vi "test2-SyncMessageWithError.vi"(8 "error in (no error)":errorcluster, 11 "TestCase in":refnum<class "testcase-CSMMessage.lvclass">) -> (0 "error out":errorcluster, 3 "TestCase out":refnum<class "testcase-CSMMessage.lvclass">)   [LabVIEW 2017, in "testcase-CSMMessage.lvclass"]
uses:
  testcase-CSMMessage.lvclass
  1ed8f569-7b65-4950-a766-51d9a6509acb.vi
  src/user.lib/_NEVSTOP/Communicable State Machine(CSM)/AdvanceAPI/CSM - Make String Arguments Safe.vi
  src/user.lib/_NEVSTOP/Communicable State Machine(CSM)/AdvanceAPI/CSM - Keywords.vi
  <vilib>/addons/_JKI Toolkits/VI Tester/TestCase.llb/TestCase.lvclass
  src/user.lib/_NEVSTOP/Communicable State Machine(CSM)/Communicable State Machine.lvlib
  C:/Program Files (x86)/National Instruments/LabVIEW 2017/vi.lib/addons/_JKI Toolkits/VI Tester/TestCase.llb/TestCase.lvclass
panel:
  out "Loopcount":i32
  out "concatenated string":string
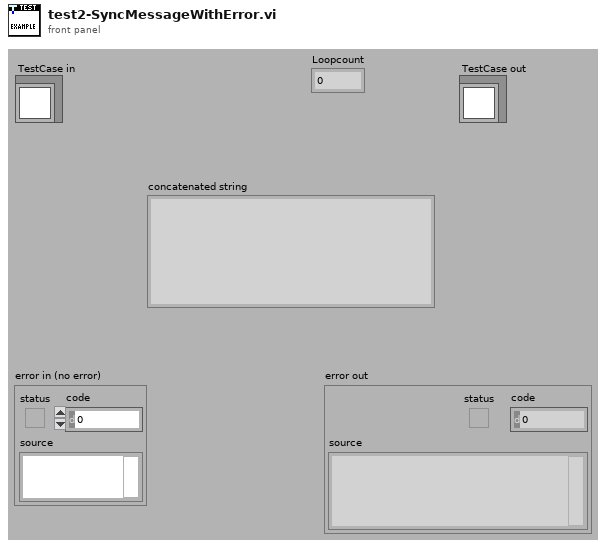
[diagram p1: front panel]
types:
  T1 = cluster{"Arguments":string, "Response":string, "error":errorcluster}
  T2 = cluster{"status":bool, "code":bool, "source":bool}
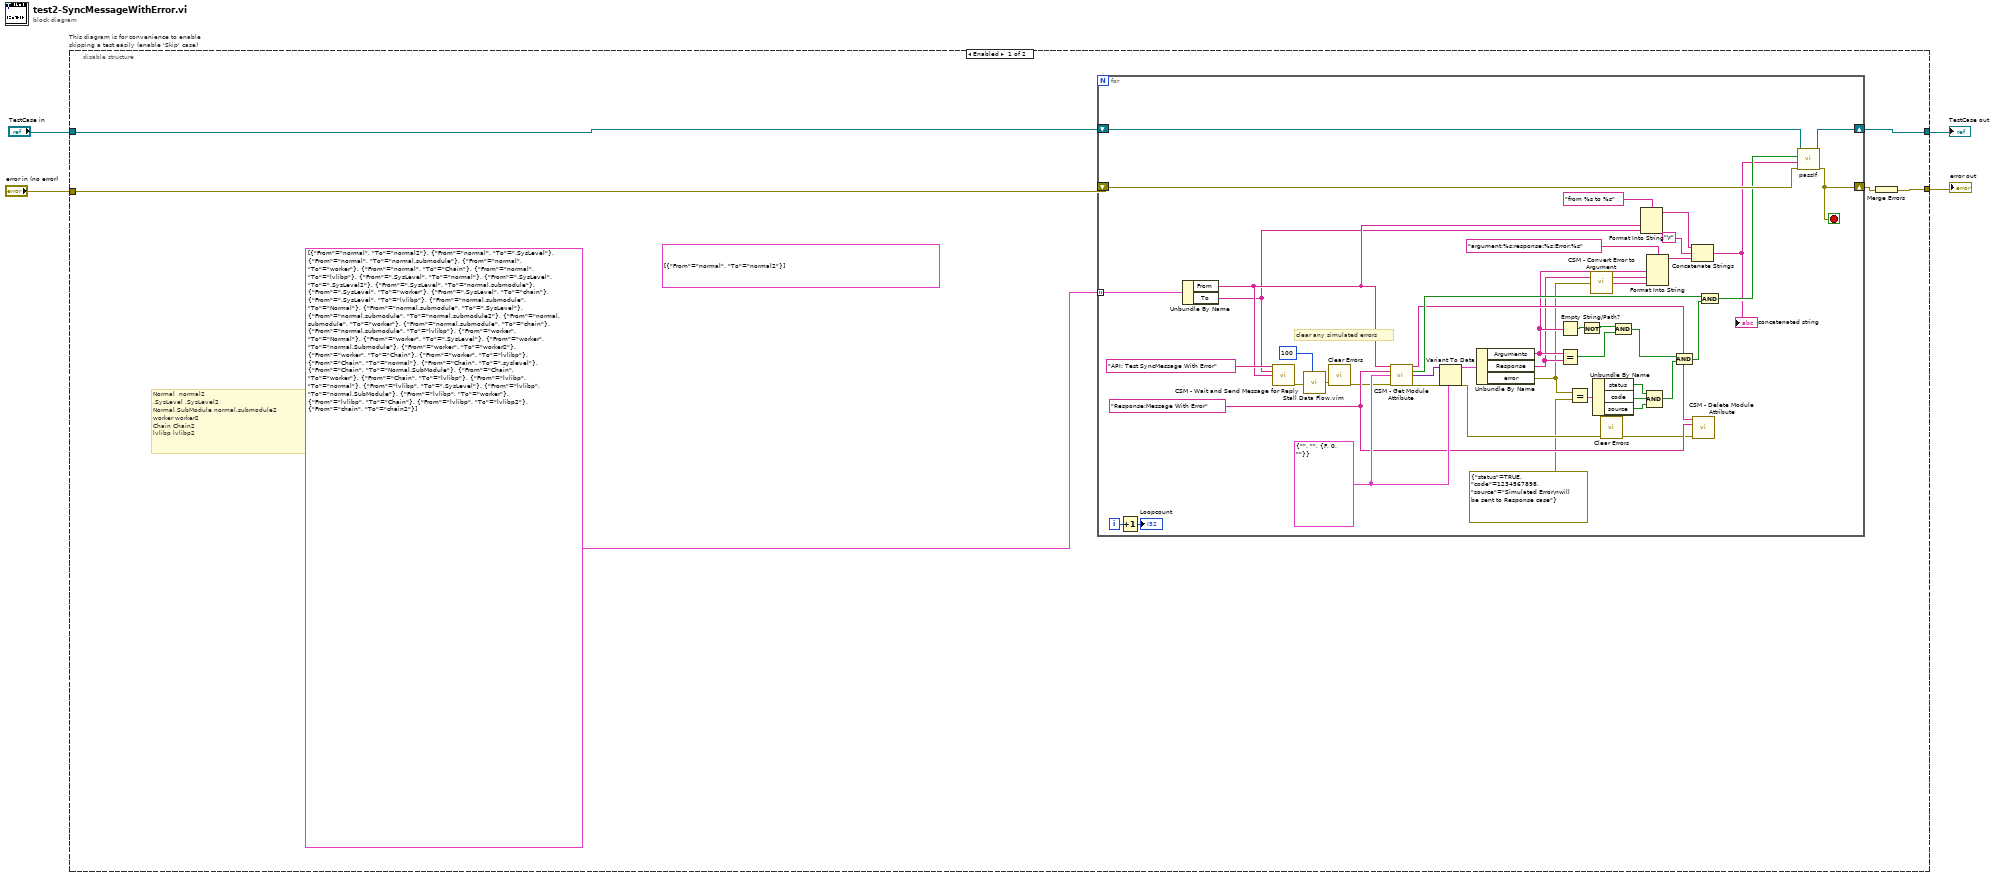
[diagram p0: block diagram]
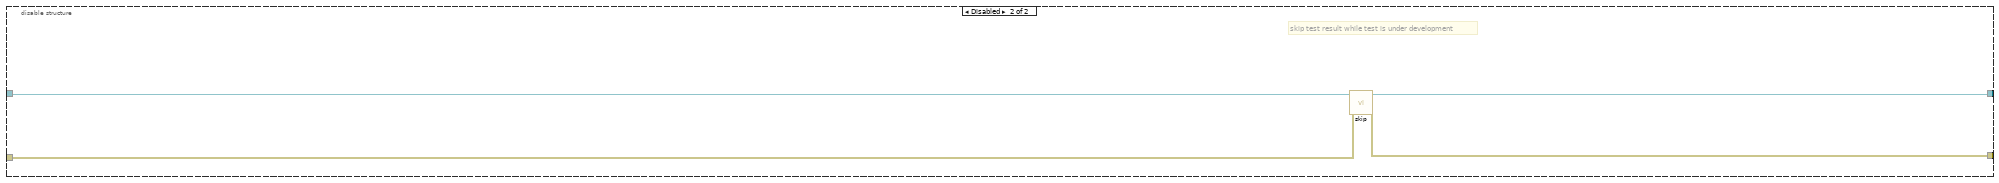
[diagram p2: hidden frame]
diagram:
  n1 = disable-structure "This diagram is for convenience to enable skipping a test easily (enable 'Skip' case)" shown="Enabled" {
    disable-tunnel: "TestCase in" -> [w10 w59]
    disable-tunnel: [w9 w57] -> w1
    disable-tunnel: [w6 w58] -> w3
    disable-tunnel: "error in (no error)" -> [w7 w56]
    frame Enabled {
      (unwired) cluster{"From":string, "To":string}[] [{"From"="normal", "To"="normal2"}]
      # "Normal  normal2\n.SysLevel .SysLevel2\nNormal.SubModule normal.submodule2\nworker worker2\nChain Chain2\nlvlibp lvlibp2"
      n2 = for {
        tunnel: cluster{"From":string, "To":string}[] [{"From"="normal", "To"="normal2"}, {"From"="normal", "To"=".SysLevel"}, {"From"="normal", "To"="normal.submodule"}, {"From"="normal", "To"="worker"}, {"From"="normal", "To"="Chain"}, {"From"="normal", "To"="lvlibp"}, {"From"=".SysLevel", "To"="normal"}, {"From"=".SysLevel", "To"=".SysLevel2"}, {"From"=".SysLevel", "To"="normal.submodule"}, {"From"=".SysLevel", "To"="worker"}, {"From"=".SysLevel", "To"="chain"}, {"From"=".SysLevel", "To"="lvlibp"}, {"From"="normal.submodule", "To"="Normal"}, {"From"="normal.submodule", "To"=".SysLevel"}, {"From"="normal.submodule", "To"="normal.submodule2"}, {"From"="normal.submodule", "To"="worker"}, {"From"="normal.submodule", "To"="chain"}, {"From"="normal.submodule", "To"="lvlibp"}, {"From"="worker", "To"="Normal"}, {"From"="worker", "To"=".SysLevel"}, {"From"="worker", "To"="normal.Submodule"}, {"From"="worker", "To"="worker2"}, {"From"="worker", "To"="Chain"}, {"From"="worker", "To"="lvlibp"}, {"From"="Chain", "To"="normal"}, {"From"="Chain", "To"=".syslevel"}, {"From"="Chain", "To"="Normal.SubModule"}, {"From"="Chain", "To"="worker"}, {"From"="Chain", "To"="lvlibp"}, {"From"="lvlibp", "To"="normal"}, {"From"="lvlibp", "To"=".SysLevel"}, {"From"="lvlibp", "To"="normal.SubModule"}, {"From"="lvlibp", "To"="worker"}, {"From"="lvlibp", "To"="Chain"}, {"From"="lvlibp", "To"="lvlibp2"}, {"From"="chain", "To"="chain2"}] -> [w44] mode=indexing
        shift-right: [w54] -> w9
        shift-left: w10 -> [w55]
        shift-right: [w26] -> w8
        shift-left: w7 -> [w53]
        i -> [w15]
        stop <- w26 stop-if-true
        w50 = T1 {"Arguments"="", "Response"="", "error"={"status"=FALSE, "code"=0, "source"=""}}
        w41 = "Response:Message With Error" ("State")
        # "clear any simulated errors"
        n3 = Increment(x=w15) -> (x+1=→"Loopcount":i32)
        n4 = Unbundle By Name(w44) -> ("From"=w17:string, "To"=w16:string)
        n5 = call "CSM - Wait and Send Message for Reply.vi"("State"="API: Test SyncMessage With Error", "Arguments (\"\")"=w16, "Target Module"=w17) -> ("error out"=w13:errorcluster)  [unwired: 10 in, 2 out]
        n6 = call "Stall Data Flow.vim"("value in"=w13, "milliseconds to wait"=u32 100) -> ("value out"=w12:errorcluster)  [unwired: 1 out]
        n7 = call <vilib>:"Clear Errors.vi"("error in (no error)"=w12) -> ("error out"=w18:errorcluster)  [unwired: 5 in, 1 out]
        n8 = call "CSM - Get Module Attribute.vi"("CSM Name"=w17, "Attribute"=w41, "Default Value (Empty Variant)"=w50, "Error In"=w18) -> ("CSM Name (Dup)"=w42:string, "Found"=w47:bool, "Value"=w49:variant, "error out"=w51:errorcluster)  [unwired: 7 in, 1 out]
        n9 = Variant To Data(error in=w51, type=w50, Variant=w49) -> (data=w48:T1, error out=w28:errorcluster)
        n10 = Unbundle By Name(w48) -> ("Arguments"=w36:string, "Response"=w35:string, "error"=w25:errorcluster)
        n11 = Empty String/Path?(string/path=w36) -> (empty?=w40:bool)
        n12 = Equal?(x=w36, y=w35) -> (x = y?=w38:bool)
        n13 = Equal?(x=w25, y=errorcluster {"status"=TRUE, "code"=1234567898, "source"="Simulated Error\nwill be sent to Response case"} ("error out")) -> (x = y?=w23:T2)
        n14 = Not(x=w40) -> (.not. x?=w39:bool)
        n15 = call "CSM - Convert Error to Argument.vi"("Error"=w25) -> ("Argument"=w34:string)  [unwired: 4 in]
        n16 = Unbundle By Name(w23) -> ("status"=w22:bool, "code"=w21:bool, "source"=w20:bool)
        n17 = call <vilib>:"Clear Errors.vi"("error in (no error)"=w28) -> ("error out"=w27:errorcluster)  [unwired: 5 in, 1 out]
        n18 = And(x=w39, y=w38) -> (x .and. y?=w37:bool)
        n19 = Format Into String(format string="from %s to %s", w17, w16) -> (resulting string=w30:string)  [unwired: 2 in, 1 out]
        n20 = Format Into String(format string="argument:%s;response:%s;Error:%s", w36, w35, w34) -> (resulting string=w33:string)  [unwired: 2 in, 1 out]
        n21 = Compound Arithmetic op=AND(w22, w21, w20) -> (w19:bool)
        n22 = And(x=w37, y=w19) -> (x .and. y?=w46:bool)
        n23 = Concatenate Strings(w30, "\r", w33) -> (w31:string)
        "concatenated string" <- w31
        n24 = call "CSM - Delete Module Attribute.vi"("CSM Name"=w42, "Attribute"=w41, "Error In"=w27) -> ()  [unwired: 9 in, 4 out]
        n25 = And(x=w47, y=w46) -> (x .and. y?=w45:bool)
        n26 = call-dynamic "passIf.vi"("error in (no error)"=w53, "message (\"\")"=w31, "pass"=w45, "TestCase in"=w55) -> ("error out"=w26:errorcluster, "TestCase out"=w54:refnum<class "testcase-CSMMessage.lvclass">)  [unwired: 6 in]
      }
      n27 = Merge Errors(w8) -> (w6:errorcluster)
    }
    frame Disabled {
      # "skip test result while test is under development"
      n28 = call <vilib>:"skip.vi"("error in (no error)"=w56, "TestCase in"=w59) -> ("error out"=w58:errorcluster, "TestCase out"=w57:refnum<class "testcase-CSMMessage.lvclass">)  [unwired: 8 in]
    }
  }
  "error out" <- w3
  "TestCase out" <- w1
